vi "Apply Ethernet Configuration.vi"(7 "Restart (T)":bool=TRUE, 8 "error in (no error)":errorcluster, 10 "Ethernet Settings":T1={"IP Address"="192.168.1.100", "TCP (Command) Port"=12345, "TCP (Command) Read Interval (ms)"=10, "UDP (Reporting) Port"=54321, "UDP (Reporting) Write Interval (ms)"=5, "UDP Data Broadcast Enable"=FALSE}, 11 "Ethernet in":refnum<class "ENET_BS1200.lvclass">) -> (0 "error out":errorcluster, 3 "Ethernet out":refnum<class "ENET_BS1200.lvclass">)   [LabVIEW 2021, in "BS120x Driver.lvlib" / "ENET_BS1200.lvclass"]
doc: "Sends the configuration updates to the Battery Simulator 1200. Changes will not be applied until after the unit is restarted. To apply multilple configuration settings in one set, set <b>Restart</b> to false on all Settings VIs except the last one.\n(c) 2019 Bloomy Controls, Inc. All rights reserved."
uses:
  ENET_BS1200.lvclass
  TypeDefs/Ethernet Settings.ctl
  <vilib>/WebDAVClient/Advanced/Get Buffer.vi
  <vilib>/WebDAVClient/Advanced/Put Buffer.vi
  ENET_BS1200.lvclass/ENET_BS1200.ctl
  <vilib>/WebDAVClient/NI_WebDAV.lvlib
  BS120x.lvclass
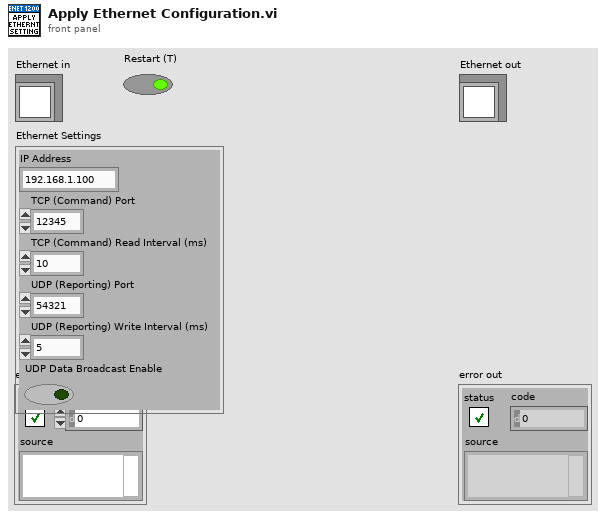
[diagram p1: front panel]
types:
  T1 = typedef "BS120x Driver.lvlib/BS120x.lvclass/Ethernet Settings.ctl" = cluster{"IP Address":string, "TCP (Command) Port":u16, "TCP (Command) Read Interval (ms)":u32, "UDP (Reporting) Port":u16, "UDP (Reporting) Write Interval (ms)":u32, "UDP Data Broadcast Enable":bool}
  T2 = typedef "NI_WebDAV.lvlib/SessionHandle.ctl" = refnum<k1>
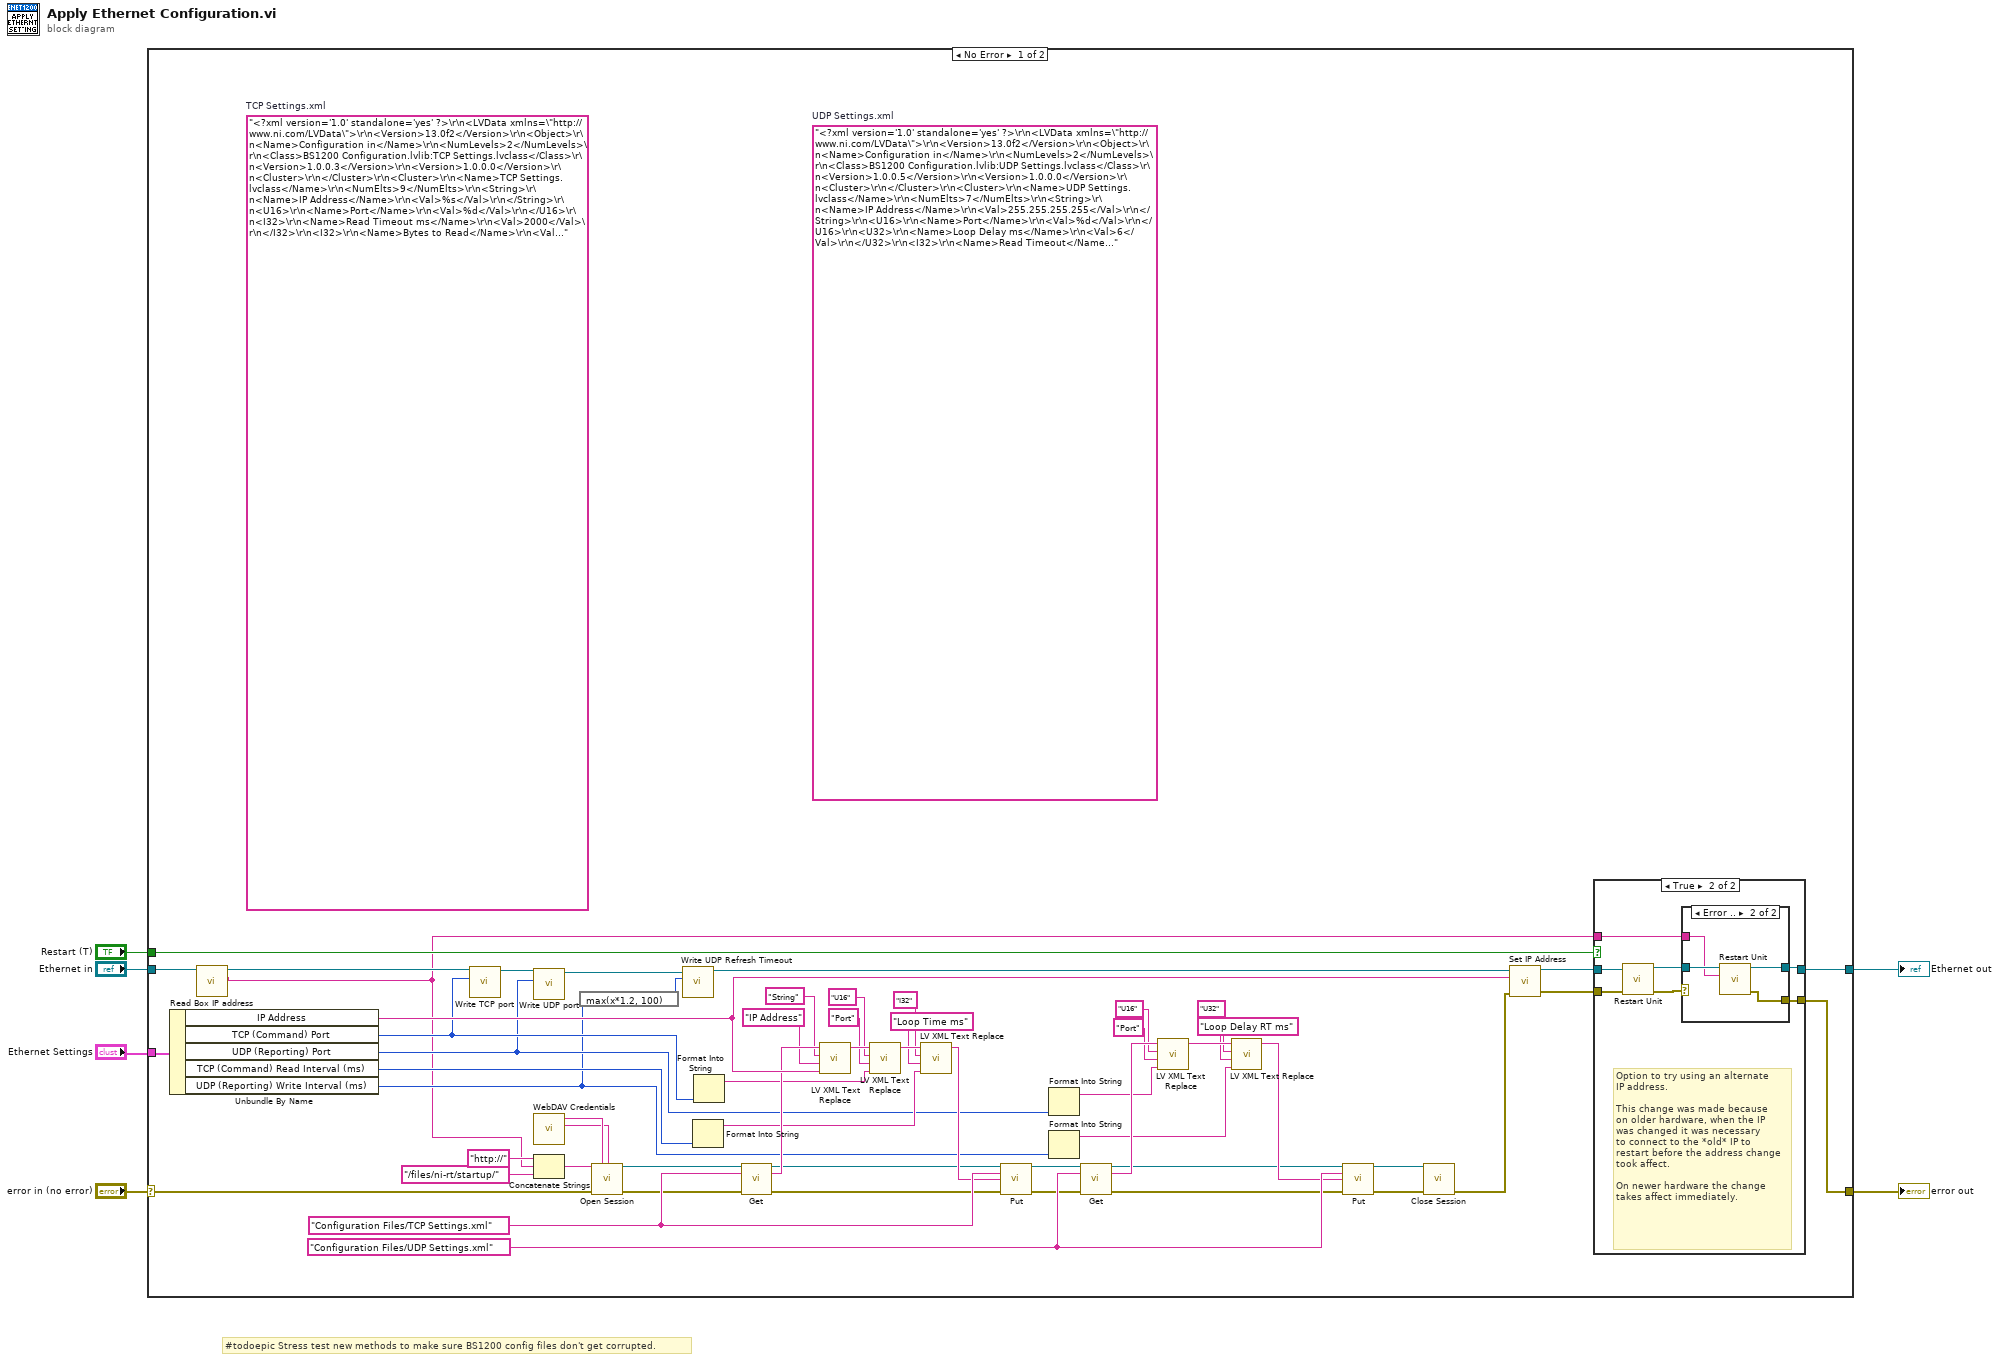
[diagram p0: block diagram]
diagram:
  # "#todoepic Stress test new methods to make sure BS1200 config files don't get corrupted."
  n1 = case shown="No Error" "error in (no error)" {
    selector: "error in (no error)" -> [w62 w81]
    tunnel: [w19 w81] -> w5
    tunnel: [w16 w80] -> w3
    tunnel: "Ethernet in" -> [w21 w80]
    tunnel: "Ethernet Settings" -> [w58 _]
    tunnel: "Restart (T)" -> [w17 _]
    frame No Error {
      (unwired) "<?xml version='1.0' standalone='yes' ?>\r\n<LVData xmlns=\"http://www.ni.com/LVData\">\r\n<Version>13.0f2</Version>\r\n<Object>\r\n<Name>Configuration in</Name>\r\n<NumLevels>2</NumLevels>\r\n<Class>BS1200 Configuration.lvlib:UDP Settings.lvclass</Class>\r\n<Version>1.0.0.5</Version>\r\n<Version>1.0.0.0</Version>\r\n<Cluster>\r\n</Cluster>\r\n<Cluster>\r\n<Name>UDP Settings.lvclass</Name>\r\n<NumElts>7</NumElts>\r\n<String>\r\n<Name>IP Address</Name>\r\n<Val>255.255.255.255</Val>\r\n</String>\r\n<U16>\r\n<Name>Port</Name>\r\n<Val>%d</Val>\r\n</U16>\r\n<U32>\r\n<Name>Loop Delay ms</Name>\r\n<Val>6</Val>\r\n</U32>\r\n<I32>\r\n<Name>Read Timeout</Name>\r\n<Val>1</Val>\r\n</I32>\r\n<I32>\r\n<Name>Max Bytes</Name>\r\n<Val>548</Val>\r\n</I32>\r\n<U32>\r\n<Name>Loop Delay RT ms</Name>\r\n<Val>%d</Val>\r\n</U32>\r\n<I32>\r\n<Name>Write Timeout</Name>\r\n<Val>0</Val>\r\n</I32>\r\n</Cluster>\r\n</Object>\r\n</LVData>"  # UDP Settings.xml
      (unwired) "<?xml version='1.0' standalone='yes' ?>\r\n<LVData xmlns=\"http://www.ni.com/LVData\">\r\n<Version>13.0f2</Version>\r\n<Object>\r\n<Name>Configuration in</Name>\r\n<NumLevels>2</NumLevels>\r\n<Class>BS1200 Configuration.lvlib:TCP Settings.lvclass</Class>\r\n<Version>1.0.0.3</Version>\r\n<Version>1.0.0.0</Version>\r\n<Cluster>\r\n</Cluster>\r\n<Cluster>\r\n<Name>TCP Settings.lvclass</Name>\r\n<NumElts>9</NumElts>\r\n<String>\r\n<Name>IP Address</Name>\r\n<Val>%s</Val>\r\n</String>\r\n<U16>\r\n<Name>Port</Name>\r\n<Val>%d</Val>\r\n</U16>\r\n<I32>\r\n<Name>Read Timeout ms</Name>\r\n<Val>2000</Val>\r\n</I32>\r\n<I32>\r\n<Name>Bytes to Read</Name>\r\n<Val>500</Val>\r\n</I32>\r\n<I32>\r\n<Name>Loop Time ms</Name>\r\n<Val>%d</Val>\r\n</I32>\r\n<I32>\r\n<Name>Primary NIC:IP Address Request Mode</Name>\r\n<Val>1</Val>\r\n</I32>\r\n<String>\r\n<Name>Subnet Mask</Name>\r\n<Val>255.255.255.0</Val>\r\n</String>\r\n<I32>\r\n<Name>Write Timeout ms</Name>\r\n<Val>5000</Val>\r\n</I32>\r\n<I32>\r\n<Name>Heartbeat Loop Time ms</Name>\r\n<Val>1000</Val>\r\n</I32>\r\n</Cluster>\r\n</Object>\r\n</LVData>"  # TCP Settings.xml
      w53 = "Configuration Files/UDP Settings.xml" ("string")
      w55 = "Configuration Files/TCP Settings.xml" ("string")
      n2 = Unbundle By Name(w58) -> ("IP Address"=w49:string, "TCP (Command) Port"=w14:u16, "UDP (Reporting) Port"=w12:u16, "TCP (Command) Read Interval (ms)"=w50:u32, "UDP (Reporting) Write Interval (ms)"=w10:u32)
      n3 = call-dynamic "Read Box IP address.vi"("ENET_BS120x in"=w21) -> ("Box IP address"=w7:string, "ENET_BS120x out"=w15:refnum<class "ENET_BS1200.lvclass">)  [unwired: 8 in, 1 out]
      n4 = call-dynamic "Write TCP port.vi"("TCP port"=w14, "ENET_BS120x in"=w15) -> ("ENET_BS120x out"=w13:refnum<class "ENET_BS1200.lvclass">)  [unwired: 8 in, 1 out]
      n5 = call-dynamic "Write UDP port.vi"("UDP port"=w12, "ENET_BS120x in"=w13) -> ("ENET_BS120x out"=w11:refnum<class "ENET_BS1200.lvclass">)  [unwired: 8 in, 1 out]
      n6 = call "WebDAV Credentials.vi"() -> ("Password"=w60:string, "Username"=w61:string)  [unwired: 10 in]
      n7 = Concatenate Strings("http://" ("string"), w7, "/files/ni-rt/startup/" ("string")) -> (w59:string)
      n8 = expression code="max(x*1.2, 100)"(w10) -> (w9:u32)
      n9 = call <vilib>:"Open Session.vi"("host uri prefix"=w59, "username"=w61, "password"=w60, "error in (no error)"=w62) -> ("session handle out"=w56:T2, "error out"=w54:errorcluster)  [unwired: 10 in]
      n10 = call-dynamic "Write UDP Refresh Timeout.vi"("UDP Refresh Timeout"=w9, "ENET_BS120x in"=w11) -> ("ENET_BS120x out"=w8:refnum<class "ENET_BS1200.lvclass">)  [unwired: 8 in, 1 out]
      n11 = Format Into String(w50) -> (resulting string=w36:string)  [unwired: 3 in, 1 out]
      n12 = Format Into String(w14) -> (resulting string=w35:string)  [unwired: 3 in, 1 out]
      n13 = call-poly <vilib>:"Get.vi"("session handle"=w56, "relative uri"=w55, "error in (no error)"=w54) -> ("session handle out"=w33:T2, "data"=w48:string, "error out"=w34:errorcluster)  [unwired: 10 in]
      n14 = call "LV XML Text Replace.vi"("Text"=w49, "Tag"="IP Address", "Datatype"="String", "LV XML in"=w48) -> ("LV XML out"=w42:string)  [unwired: 7 in]
      n15 = call "LV XML Text Replace.vi"("Text"=w35, "Tag"="Port", "Datatype"="U16", "LV XML in"=w42) -> ("LV XML out"=w41:string)  [unwired: 7 in]
      n16 = call "LV XML Text Replace.vi"("Text"=w36, "Tag"="Loop Time ms", "Datatype"="I32", "LV XML in"=w41) -> ("LV XML out"=w47:string)  [unwired: 7 in]
      n17 = call-poly <vilib>:"Put.vi"("session handle"=w33, "relative uri"=w55, "data"=w47, "error in (no error)"=w34) -> ("session handle out"=w31:T2, "error out"=w32:errorcluster)  [unwired: 10 in]
      n18 = Format Into String(w12) -> (resulting string=w25:string)  [unwired: 3 in, 1 out]
      n19 = Format Into String(w10) -> (resulting string=w24:string)  [unwired: 3 in, 1 out]
      n20 = call-poly <vilib>:"Get.vi"("session handle"=w31, "relative uri"=w53, "error in (no error)"=w32) -> ("session handle out"=w22:T2, "data"=w46:string, "error out"=w23:errorcluster)  [unwired: 10 in]
      n21 = call "LV XML Text Replace.vi"("Text"=w25, "Tag"="Port", "Datatype"="U16", "LV XML in"=w46) -> ("LV XML out"=w30:string)  [unwired: 7 in]
      n22 = call "LV XML Text Replace.vi"("Text"=w24, "Tag"="Loop Delay RT ms", "Datatype"="U32", "LV XML in"=w30) -> ("LV XML out"=w45:string)  [unwired: 7 in]
      n23 = call-poly <vilib>:"Put.vi"("session handle"=w22, "relative uri"=w53, "data"=w45, "error in (no error)"=w23) -> ("session handle out"=w51:T2, "error out"=w52:errorcluster)  [unwired: 10 in]
      n24 = call <vilib>:"Close Session.vi"("session handle"=w51, "error in (no error)"=w52) -> ("error out"=w57:errorcluster)  [unwired: 13 in]
      n25 = call-dynamic "Set IP Address.vi"("error in (no error)"=w57, "IP Address"=w49, "ENET in"=w8) -> ("error out"=w20:errorcluster, "ENET out"=w18:refnum<class "ENET_BS1200.lvclass">)  [unwired: 7 in]
      n26 = case shown="True" w17 {
        tunnel: w20 -> [w66 w73]
        tunnel: [w66 w67] -> w19
        tunnel: w18 -> [w65 w72]
        tunnel: [w65 w70] -> w16
        tunnel: w7 -> [_ w68]
        frame False {
        }
        frame True {
          # "Option to try using an alternate\nIP address.\n\nThis change was made because\non older hardware, when the IP\nwas changed it was necessary\nto connect to the *old* IP to\nrestart before the address change\ntook affect.\n\nOn newer hardware the change\ntakes affect immediately."
          n27 = call-dynamic "Restart Unit.vi"("error in (no error)"=w73, "ENET in"=w72) -> ("error out"=w69:errorcluster, "ENET out"=w71:refnum<class "ENET_BS1200.lvclass">)  [unwired: 8 in]
          n28 = case shown="Error .." w69 {
            selector: w69 -> [w74 _]
            tunnel: w71 -> [w75 w79]
            tunnel: [w75 w78] -> w70
            tunnel: w68 -> [_ w77]
            tunnel: [w74 w76] -> w67
            frame No Error {
            }
            frame Error {
              n29 = call-dynamic "Restart Unit.vi"("New IP (empty = original)"=w77, "ENET in"=w79) -> ("error out"=w76:errorcluster, "ENET out"=w78:refnum<class "ENET_BS1200.lvclass">)  [unwired: 8 in]
            }
          }
        }
      }
    }
    frame Error {
    }
  }
  "error out" <- w5
  "Ethernet out" <- w3
